vi "Instr_InitObject.vi"(8 "error in (no error)":errorcluster, 9 "Instrument Configuration":variant, 10 "GPIB Address":string, 11 "GPIBSwitching in":refnum<class "GPIBSwitching.lvclass">) -> (0 "error out":errorcluster, 3 "GPIBSwitching out":refnum<class "GPIBSwitching.lvclass">)   [LabVIEW 2018, in "GPIBSwitching.lvclass"]
uses:
  GPIBSwitching.lvclass
  InstrumentSetup.vi
  MUX_CommandsGlobal.vi
  Matrix_CommandsGlobal.vi
  InstrControl.lvclass
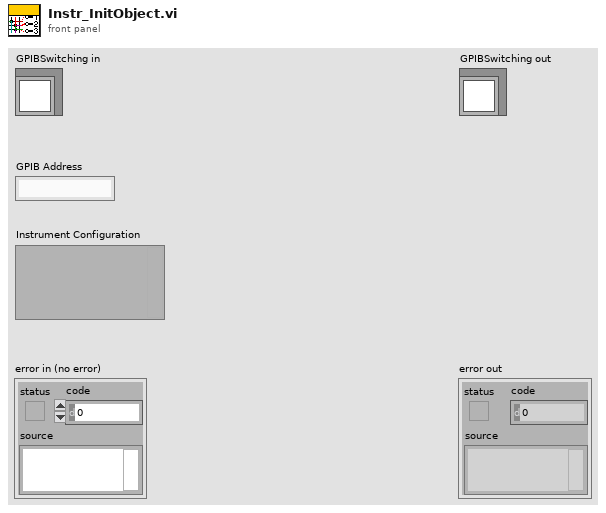
[diagram p1: front panel]
types:
  T1 = cluster{"Matrix address":string, "Mux1 address":string, "Mux2 address":string, "Matrix used?":bool, "Switching":refnum<class "Switching.lvclass">, "Matrix X Channels":cluster{"Bias Supply / SMU LO":i32, "Bias Supply / SMU HI":i32, "CV Box LO":i32, "CV Box HI":i32, "CV Box LO IN":i32, "CV Box HI IN":i32, "Volt meter LO":i32, "Volt meter HI":i32, "Mux1 C1":i32, "Mux1 C2":i32, "Mux2 C1":i32, "Mux2 C2":i32}}
  T2 = cluster{"Matrix address":string, "Instrument name":string, "Instrument type":u16, "Command \"Matrix Reset\"":string, "Command \"Connect Matrix Channels\"":string, "Command \"Disconnect Matrix Channels\"":string}
  T3 = cluster{"Mux1 address":string, "Mux2 address":string, "Instrument name":string, "Instrument type":u16, "Command \"MUX Reset\"":string, "Command \"Select MUX Channel\"":string}
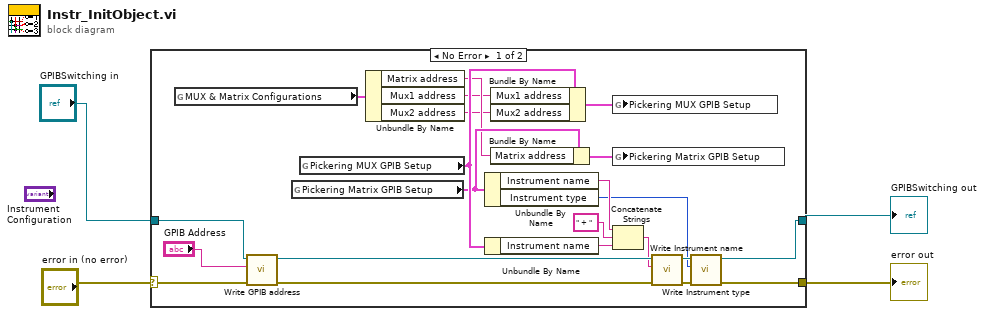
[diagram p0: block diagram]
diagram:
  n1 = case shown="No Error" "error in (no error)" {
    selector: "error in (no error)" -> [w21 w28]
    tunnel: [w14 w28] -> w2
    tunnel: "GPIBSwitching in" -> [w20 w27]
    tunnel: [w13 w27] -> w3
    frame No Error {
      n2 = global read "InstrumentSetup.vi" "MUX & Matrix Configurations"() -> (w26:T1)
      n3 = call-dynamic "Write GPIB address.vi"("error in (no error)"=w21, "GPIB address"="GPIB Address", "InstControl in"=w20) -> ("error out"=w23:errorcluster, "InstControl out"=w25:refnum<class "GPIBSwitching.lvclass">)  [unwired: 7 in]
      n4 = global read "Matrix_CommandsGlobal.vi" "Pickering Matrix GPIB Setup"() -> (w11:T2)
      n5 = global read "MUX_CommandsGlobal.vi" "Pickering MUX GPIB Setup"() -> (w12:T3)
      n6 = Unbundle By Name(w26) -> ("Matrix address"=w10:string, "Mux1 address"=w9:string, "Mux2 address"=w8:string)
      n7 = Unbundle By Name(w11) -> ("Instrument name"=w19:string, "Instrument type"=w15:u16)
      n8 = Unbundle By Name(w12) -> ("Instrument name"=w18:string)
      n9 = Bundle By Name(cluster=w12, "Mux1 address"=w9, "Mux2 address"=w8) -> (w7:T3)
      n10 = Bundle By Name(cluster=w11, "Matrix address"=w10) -> (w6:T2)
      n11 = global write "MUX_CommandsGlobal.vi" "Pickering MUX GPIB Setup"(w7) -> ()
      n12 = global write "Matrix_CommandsGlobal.vi" "Pickering Matrix GPIB Setup"(w6) -> ()
      n13 = Concatenate Strings(w19, " + ", w18) -> (w16:string)
      n14 = call-dynamic "Write Instrument name.vi"("error in (no error)"=w23, "Instrument name"=w16, "InstControl in"=w25) -> ("error out"=w22:errorcluster, "InstControl out"=w24:refnum<class "GPIBSwitching.lvclass">)  [unwired: 7 in]
      n15 = call-dynamic "Write Instrument type.vi"("error in (no error)"=w22, "Instrument type"=w15, "InstControl in"=w24) -> ("error out"=w14:errorcluster, "InstControl out"=w13:refnum<class "GPIBSwitching.lvclass">)  [unwired: 7 in]
    }
    frame Error {
    }
  }
  "error out" <- w2
  "GPIBSwitching out" <- w3
